vi "Display Channel MUX.vi"(0 "tagged llp packets cluster":T1, 1 "reset":bool, 2 "pending display frames":i8, 5 "display parameters in":T11[](array[typedef])=[{"virtual channel"=0.0, "payload data type"=enum."Frame Start", "frame skip count"=0, "line skip count"=0, "pixel skip count"=0.0}, {"virtual channel"=0.0, "payload data type"=enum."Frame Start", "frame skip count"=0, "line skip count"=0, "pixel skip count"=0.0}, {"virtual channel"=0.0, "payload data type"=enum."Frame Start", "frame skip count"=0, "line skip count"=0, "pixel skip count"=0.0}, {"virtual channel"=0.0, "payload data type"=enum."Frame Start", "frame skip count"=0, "line skip count"=0, "pixel skip count"=0.0}, {"virtual channel"=0.0, "payload data type"=enum."Frame Start", "frame skip count"=0, "line skip count"=0, "pixel skip count"=0.0}, {"virtual channel"=0.0, "payload data type"=enum."Frame Start", "frame skip count"=0, "line skip count"=0, "pixel skip count"=0.0}, {"virtual channel"=0.0, "payload data type"=enum."Frame Start", "frame skip count"=0, "line skip count"=0, "pixel skip count"=0.0}, {"virtual channel"=0.0, "payload data type"=enum."Frame Start", "frame skip count"=0, "line skip count"=0, "pixel skip count"=0.0}], 7 "channel selector":fxp<+,3,3>, 9 "input valid":bool[](array[boolean])=[FALSE, FALSE, FALSE, FALSE, FALSE, FALSE, FALSE, FALSE], 12 "ready for output":bool) -> (3 "clear processing pipeline":bool, 4 "llp packet out":T7, 6 "display parameters out":T11, 8 "selected channel":fxp<+,3,3>, 10 "output valid":bool, 14 "ready for input":bool)   [LabVIEW 2020, in "GettingStarted_Common_148X_FPGA.lvlib"]
uses:
  GettingStarted_Common_148X_FPGA.lvlib
  <instrlib>/FlexRIO/CSI-2/v2/FPGA/Types/Display Parameters.ctl
  <instrlib>/FlexRIO/CSI-2/v2/Common/Types/LLP Data Type.ctl
  <instrlib>/FlexRIO/CSI-2/v2/FPGA/Types/LLP Packet.ctl
  <instrlib>/FlexRIO/CSI-2/v2/FPGA/Types/LLP Packet Header.ctl
  <instrlib>/FlexRIO/CSI-2/v2/FPGA/Types/LLP Packet Payload.ctl
  <instrlib>/FlexRIO/CSI-2/v2/FPGA/Types/LLP Packet Footer.ctl
  Types/Tagged LLP Packets Cluster.ctl
  <instrlib>/FlexRIO/CSI-2/v2/FPGA/Types/Tagged LLP Packet.ctl
  <instrlib>/FlexRIO/CSI-2/v2/FPGA/Types/FPGA LLP Packet Tag.ctl
  <instrlib>/FlexRIO/CSI-2/v2/FPGA/Types/FPGA LLP Packet Timestamp.ctl
  <instrlib>/FlexRIO/CSI-2/v2/FPGA/Types/Timestamp ID.ctl
  <instrlib>/FlexRIO/CSI-2/v2/FPGA/Types/FPGA LLP Packet Size.ctl
  Types/Display Channel MUX State Data.ctl
  Types/Display Channel MUX State.ctl
  8cc59fb1-aa29-4151-ba24-7106bc360e93.vi
  <instrlib>/FlexRIO/CSI-2/v2/FPGA/NI CSI-2 API FPGA v2.lvlib
  <instrlib>/FlexRIO/CSI-2/v2/Common/NI CSI-2 API Common v2.lvlib
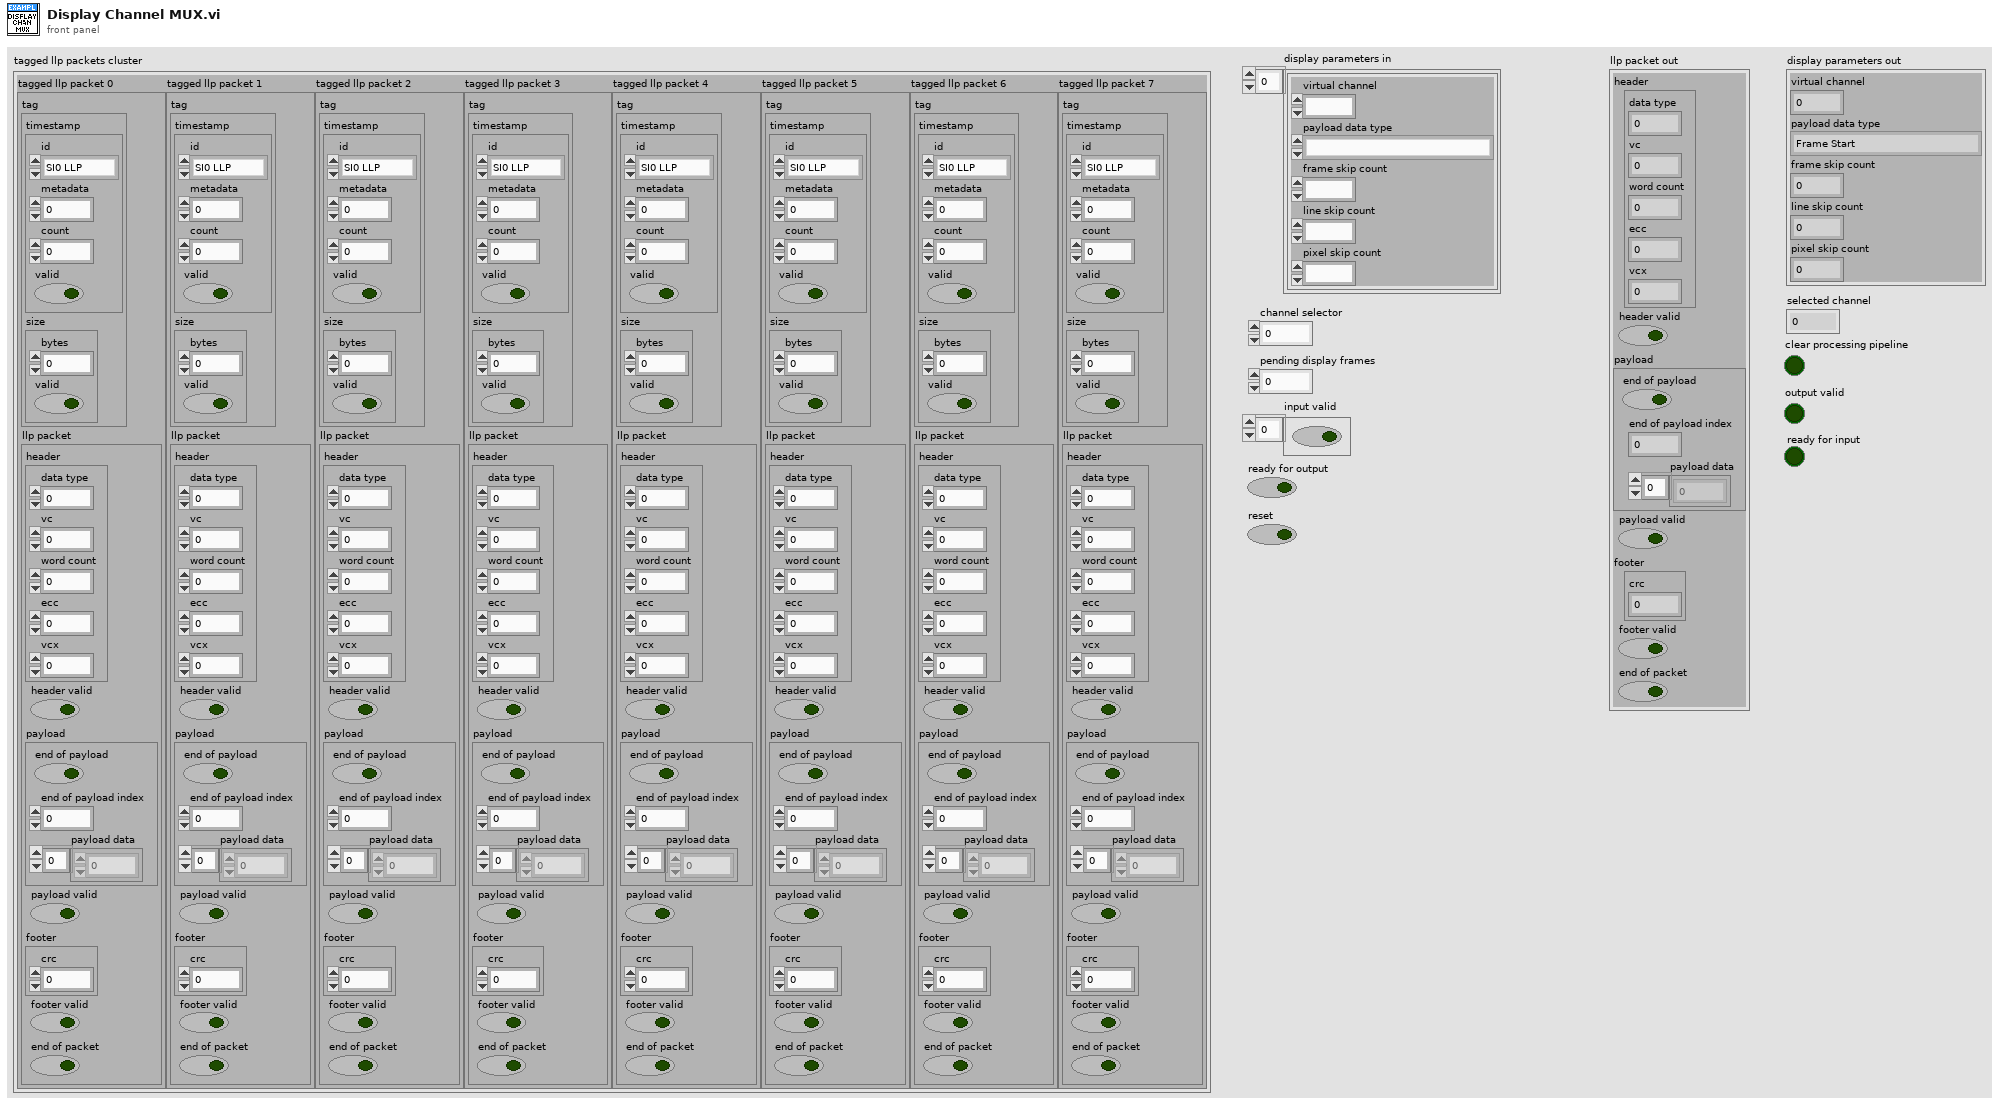
[diagram p1: front panel]
types:
  T1 = typedef "GettingStarted_Common_148X_FPGA.lvlib/Tagged LLP Packets Cluster.ctl" = cluster{"tagged llp packet 0":T2, "tagged llp packet 1":T2, "tagged llp packet 2":T2, "tagged llp packet 3":T2, "tagged llp packet 4":T2, "tagged llp packet 5":T2, "tagged llp packet 6":T2, "tagged llp packet 7":T2}
  T2 = typedef "NI CSI-2 API FPGA v2.lvlib/Tagged LLP Packet.ctl" = cluster{"tag":T3, "llp packet":T7}
  T3 = typedef "NI CSI-2 API FPGA v2.lvlib/FPGA LLP Packet Tag.ctl" = cluster{"timestamp":T4, "size":T6}
  T4 = typedef "NI CSI-2 API FPGA v2.lvlib/FPGA LLP Packet Timestamp.ctl" = cluster{"valid":bool, "count":fxp<+,50,50>, "id":T5, "metadata":u8}
  T5 = typedef "NI CSI-2 API FPGA v2.lvlib/Timestamp ID.ctl" = enum8{"SI0 LLP", "SI1 LLP", "SI2 LLP", "SI3 LLP", "SI4 LLP", "SI5 LLP", "SI6 LLP", "SI7 LLP", "SO0 LLP", "SO1 LLP", "SO2 LLP", "SO3 LLP", "SO4 LLP", "SO5 LLP", "SO6 LLP", "SO7 LLP", "Ser0 GPIO Bank", "Ser1 GPIO Bank", "Ser2 GPIO Bank", "Ser3 GPIO Bank", "Ser4 GPIO Bank", "Ser5 GPIO Bank", "Ser6 GPIO Bank", "Ser7 GPIO Bank", "Des0 GPIO Bank", "Des1 GPIO Bank", "Des2 GPIO Bank", "Des3 GPIO Bank", "Des4 GPIO Bank", "Des5 GPIO Bank", "Des6 GPIO Bank", "Des7 GPIO Bank", "User0", "User1", "User2", "User3", "User4", "User5", "User6", "User7", "User8", "User9", "User10", "User11", "User12", "User13", "User14", "User15", "User16", "User17", "User18", "User19", "User20", "User21", "User22", "User23", "User24", "User25", "User26", "User27", "User28", "User29", "User30", "User31"}
  T6 = typedef "NI CSI-2 API FPGA v2.lvlib/FPGA LLP Packet Size.ctl" = cluster{"bytes":fxp<+,17,17>, "valid":bool}
  T7 = typedef "NI CSI-2 API FPGA v2.lvlib/LLP Packet.ctl" = cluster{"header":T8, "header valid":bool, "payload":T9, "payload valid":bool, "footer":T10, "footer valid":bool, "end of packet":bool}
  T8 = typedef "NI CSI-2 API FPGA v2.lvlib/LLP Packet Header.ctl" = cluster{"word count":u16, "ecc":fxp<+,6,6>, "vcx":fxp<+,2,2>, "data type":fxp<+,6,6>, "vc":fxp<+,2,2>}
  T9 = typedef "NI CSI-2 API FPGA v2.lvlib/LLP Packet Payload.ctl" = cluster{"end of payload":bool, "end of payload index":fxp<+,3,3>, "payload data":u8[]}
  T10 = typedef "NI CSI-2 API FPGA v2.lvlib/LLP Packet Footer.ctl" = cluster{"crc":u16}
  T11 = typedef "NI CSI-2 API FPGA v2.lvlib/Display Parameters.ctl" = cluster{"virtual channel":fxp<+,4,4>, "payload data type":T12, "frame skip count":u16, "line skip count":u8, "pixel skip count":fxp<+,5,5>}
  T12 = typedef "NI CSI-2 API Common v2.lvlib/LLP Data Type.ctl" = enum8{"Frame Start", "Frame End", "Line Start", "Line End", "End of Transmission", "Reserved 0", "Reserved 1", "Reserved 2", "Generic Short Packet 1", "Generic Short Packet 2", "Generic Short Packet 3", "Generic Short Packet 4", "Generic Short Packet 5", "Generic Short Packet 6", "Generic Short Packet 7", "Generic Short Packet 8", "Null", "Blanking Data", "Embedded 8-bit non Image Data", "Generic Long Packet 1", "Generic Long Packet 2", "Generic Long Packet 3", "Generic Long Packet 4", "Reserved 3", "YUV420 8-bit", "YUV420 10-bit", "Legacy YUV420 8-bit", "Reserved 4", "YUV420 8-bit Chroma Shifted", "YUV420 10-bit Chroma Shifted", "YUV422 8-bit", "YUV422 10-bit", "RGB444", "RGB555", "RGB565", "RGB666", "RGB888", "Reserved 5", "Reserved 6", "RAW 24", "RAW 6", "RAW 7", "RAW 8", "RAW 10", "RAW 12", "RAW 14", "RAW 16", "RAW 20", "User Defined 8-bit Data 1", "User Defined 8-bit Data 2", "User Defined 8-bit Data 3", "User Defined 8-bit Data 4", "User Defined 8-bit Data 5", "User Defined 8-bit Data 6", "User Defined 8-bit Data 7", "User Defined 8-bit Data 8", "USL Command", "Reserved 7", "Reserved 8", "Reserved 9", "Reserved 10", "Reserved 11", "Reserved 12", "LRTE EPD Spacer"}
  T13 = typedef "GettingStarted_Common_148X_FPGA.lvlib/Display Channel MUX State.ctl" = enum8{"wait for frame start", "wait for frame end", "clear pipeline and latch settings"}
  T14 = typedef "GettingStarted_Common_148X_FPGA.lvlib/Display Channel MUX State Data.ctl" = cluster{"state":T13, "channel selector":fxp<+,3,3>, "display parameters":T11}
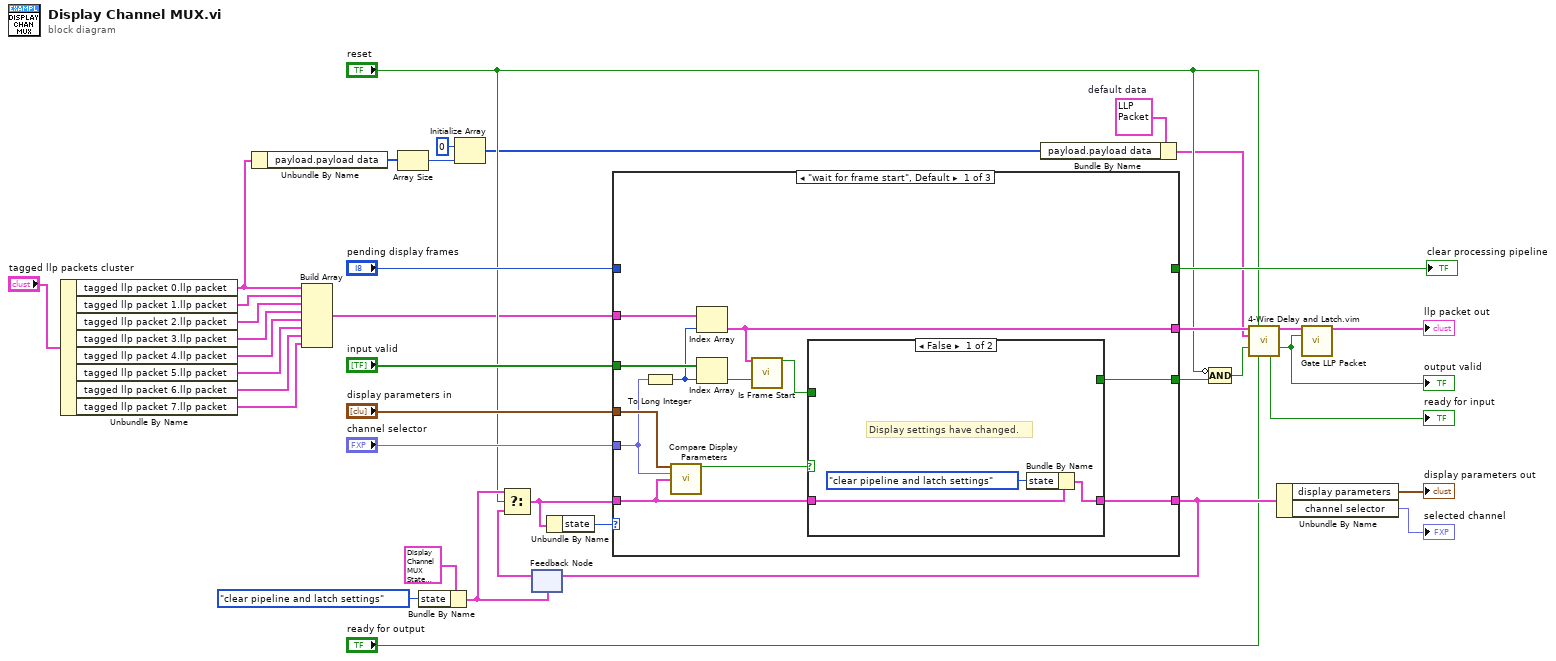
[diagram p0: block diagram]
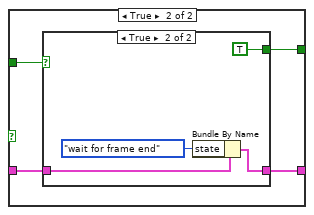
[diagram p2: hidden frame]
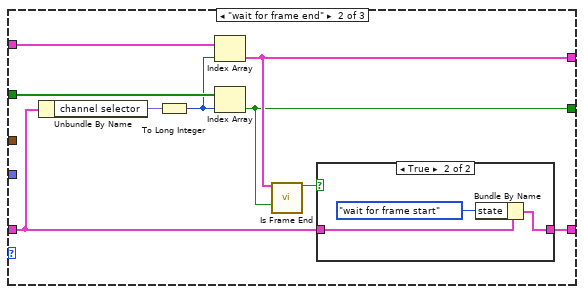
[diagram p4: hidden frame]
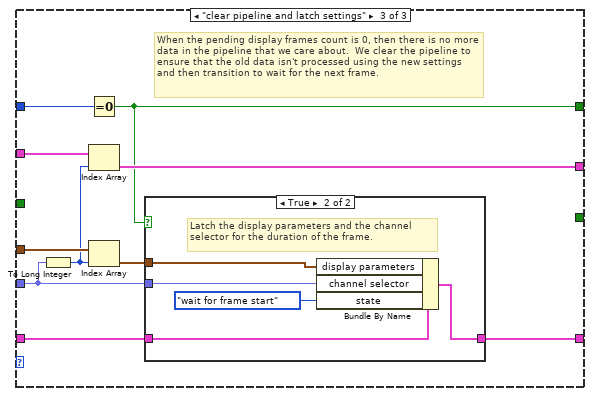
[diagram p6: hidden frame]
diagram:
  w3 = T7 {"header"={"word count"=0, "ecc"=0.0, "vcx"=0.0, "data type"=0.0, "vc"=0.0}, "header valid"=FALSE, "payload"={"end of payload"=FALSE, "end of payload index"=0.0, "payload data"=[]}, "payload valid"=FALSE, "footer"={"crc"=0}, "footer valid"=FALSE, "end of packet"=FALSE}  # default data
  n1 = Unbundle By Name("tagged llp packets cluster") -> ("tagged llp packet 0.llp packet"=w7:T7, "tagged llp packet 1.llp packet"=w10:T7, "tagged llp packet 2.llp packet"=w11:T7, "tagged llp packet 3.llp packet"=w12:T7, "tagged llp packet 4.llp packet"=w13:T7, "tagged llp packet 5.llp packet"=w14:T7, "tagged llp packet 6.llp packet"=w15:T7, "tagged llp packet 7.llp packet"=w16:T7)
  n2 = Unbundle By Name(w7) -> ("payload.payload data"=w6:u8[])
  n3 = Build Array(w7, w10, w11, w12, w13, w14, w15, w16) -> (w9:T7[])
  n4 = Array Size(array=w6) -> (size(s)=w5:i32)
  n5 = Bundle By Name(cluster=T14 {"state"=enum."wait for frame end", "channel selector"=0.0, "display parameters"={"virtual channel"=0.0, "payload data type"=enum."Frame Start", "frame skip count"=0, "line skip count"=0, "pixel skip count"=0.0}}, "state"=Display_Channel_MUX_State."clear pipeline and latch settings") -> (w33:T14)
  n6 = Initialize Array(u8 0 ("element"), w5) -> (w1:u8[])
  n7 = feedback #1(w33) -> (w34:T14)
  n8 = Select(t=w33, s="reset", f=w34) -> (s? t:f=w35:T14)
  n9 = Unbundle By Name(w35) -> ("state"=w37:T13)
  n10 = case shown="\"wait for frame start\", Default" w37 {
    tunnel: w9 -> [w51 w72 w86]
    tunnel: "input valid" -> [w50 w71 _]
    tunnel: [w46 w67 _] -> w29
    tunnel: [w44 w68 w85] -> w23
    tunnel: w35 -> [w42 w64 w83]
    tunnel: [w47 w70 w82] -> w28
    tunnel: "channel selector" -> [w41 _ w79]
    tunnel: "display parameters in" -> [w43 _ w80]
    tunnel: "pending display frames" -> [_ _ w84]
    tunnel: [_ _ w81] -> w24
    frame "wait for frame start", Default {
      n11 = To Long Integer(number=w41) -> (32bit integer=w45:i32)
      n12 = call "Compare Display Parameters.vi"("display parameters in"=w43, "channel selector"=w41, "current state"=w42) -> ("equal"=w40:bool)  [unwired: 12 in]
      n13 = Index Array(array=w51, index=w45) -> (element=w44:T7)
      n14 = Index Array(array=w50, index=w45) -> (element=w49:bool)
      n15 = call <instrlib>:"Is Frame Start.vi"("llp packet"=w44, "input valid"=w49) -> ("frame start"=w48:bool)  [unwired: 13 in]
      n16 = case shown="False" w40 {
        tunnel: w48 -> [_ w58]
        tunnel: [w54 w57] -> w47
        tunnel: [_ w56] -> w46
        tunnel: w42 -> [w53 w55]
        frame False {
          # "Display settings have changed."
          n17 = Bundle By Name(cluster=w53, "state"=Display_Channel_MUX_State."clear pipeline and latch settings") -> (w54:T14)
        }
        frame True {
          n18 = case shown="True" w58 {
            tunnel: w55 -> [w59 w63]
            tunnel: [w59 w62] -> w57
            tunnel: [_ TRUE] -> w56
            frame False {
            }
            frame True {
              n19 = Bundle By Name(cluster=w63, "state"=Display_Channel_MUX_State."wait for frame end") -> (w62:T14)
            }
          }
        }
      }
    }
    frame "wait for frame end" {
      n20 = Unbundle By Name(w64) -> ("channel selector"=w66:fxp<+,3,3>)
      n21 = To Long Integer(number=w66) -> (32bit integer=w65:i32)
      n22 = Index Array(array=w72, index=w65) -> (element=w68:T7)
      n23 = Index Array(array=w71, index=w65) -> (element=w67:bool)
      n24 = call <instrlib>:"Is Frame End.vi"("llp packet"=w68, "input valid"=w67) -> ("frame end"=w69:bool)  [unwired: 13 in]
      n25 = case shown="True" w69 {
        tunnel: w64 -> [w73 w76]
        tunnel: [w73 w75] -> w70
        frame False {
        }
        frame True {
          n26 = Bundle By Name(cluster=w76, "state"=Display_Channel_MUX_State."wait for frame start") -> (w75:T14)
        }
      }
    }
    frame "clear pipeline and latch settings" {
      # "When the pending display frames count is 0, then there is no more data in the pipeline that we care about.  We clear the pipeline to ensure that the old data isn't processed using the new settings and then transition to wait for the next frame."
      n27 = To Long Integer(number=w79) -> (32bit integer=w77:i32)
      n28 = Equal To 0?(x=w84) -> (x = 0?=w81:bool)
      n29 = Index Array(array=w86, index=w77) -> (element=w85:T7)
      n30 = Index Array(array=w80, index=w77) -> (element=w78:T11)
      n31 = case shown="True" w81 {
        tunnel: w83 -> [w87 w92]
        tunnel: [w87 w91] -> w82
        tunnel: w79 -> [_ w90]
        tunnel: w78 -> [_ w89]
        frame False {
        }
        frame True {
          # "Latch the display parameters and the channel selector for the duration of the frame."
          n32 = Bundle By Name(cluster=w92, "display parameters"=w89, "channel selector"=w90, "state"=Display_Channel_MUX_State."wait for frame start") -> (w91:T14)
        }
      }
    }
  }
  "clear processing pipeline" <- w24
  n33 = feedback-in #1(w28) -> ()
  n34 = Bundle By Name(cluster=w3, "payload.payload data"=w1) -> (w2:T7)
  n35 = Compound Arithmetic op=AND(invert "reset", w29) -> (w20:bool)
  n36 = call "4-Wire Delay and Latch.vim"("data in"=w23, "reset"="reset", "default data"=w2, "input valid"=w20, "ready for output"="ready for output") -> ("data out"=w22:T7, "output valid"=w21:bool, "ready for input"=→"ready for input":bool)  [unwired: 8 in]
  "output valid" <- w21
  n37 = Unbundle By Name(w28) -> ("display parameters"=→"display parameters out":T11, "channel selector"=→"selected channel":fxp<+,3,3>)
  n38 = call <instrlib>:"Gate LLP Packet.vi"("llp packet in"=w22, "enable"=w21) -> ("llp packet out"=→"llp packet out":T7)  [unwired: 13 in]
